vi "34970A Trigger+Read SW Scan v7.vi"(0 "VISA session":refnum<visa-resource-name>, 11 "error in":errorcluster, 12 "# Chan/Scan":i32, 13 "Error Query?":bool, 14 "Read delay mS":u32=1000) -> (4 "VISA out":refnum<visa-resource-name>, 6 "Strings":string[](array[string]), 8 "Pressures":T1, 10 "DBL":dbl[](array[numeric]) format="%.2f", 15 "error":errorcluster)   [LabVIEW 2020]
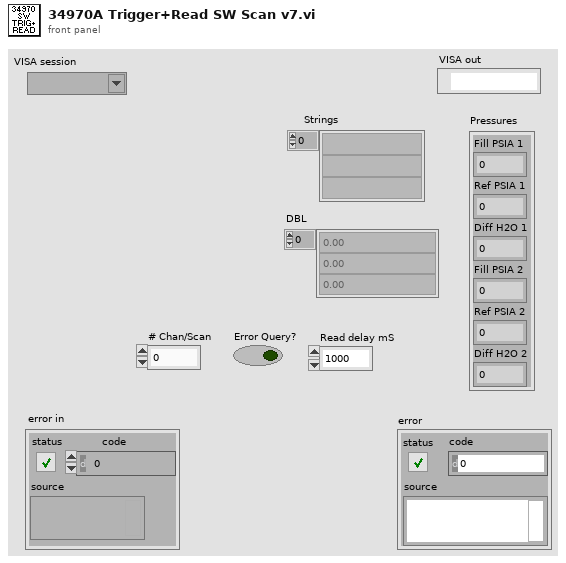
[diagram p1: front panel]
types:
  T1 = cluster{"Fill PSIA 1":dbl, "Ref PSIA 1":dbl, "Diff H2O 1":dbl, "Fill PSIA 2":dbl, "Ref PSIA 2":dbl, "Diff H2O 2":dbl}
  T2 = enum16{"Remote Trigger", "Immediate Trigger", "Wait for Trigger", "Abort Scan"}
  T3 = cluster{"Output Number Array[0]":dbl, "Output Number Array[1]":dbl, "Output Number Array[2]":dbl, "Output Number Array[3]":dbl, "Output Number Array[4]":dbl, "Output Number Array[5]":dbl}
  T4 = cluster{"Output Number Array[0]":dbl, "Output Number Array[1]":dbl, dbl, "Output Number Array[3]":dbl, "Output Number Array[4]":dbl, dbl}
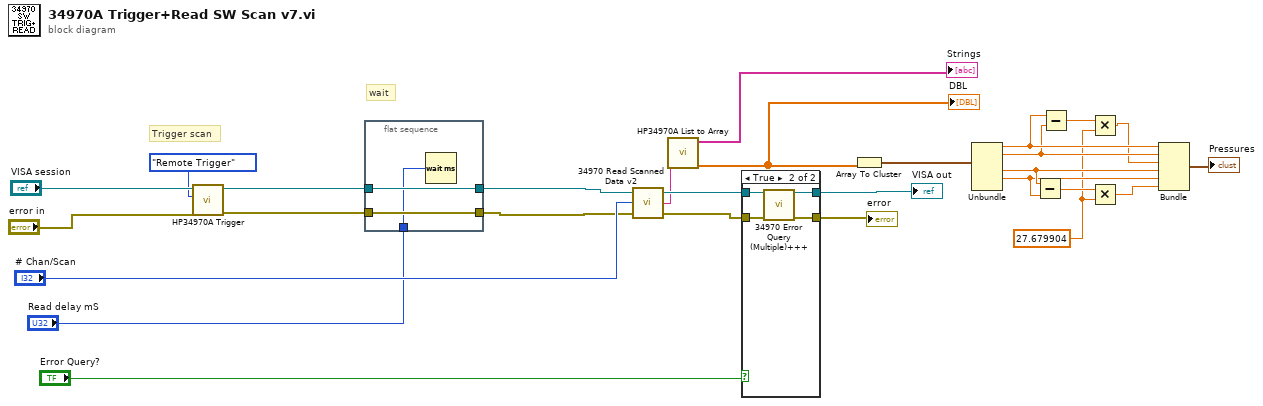
[diagram p0: block diagram]
diagram:
  w7 = 27.679904
  # "wait"
  # "Trigger scan"
  n1 = call "HP34970A Trigger.vi"("error in (no error)"="error in", "Command (0:Rem Trig)"=T2."Remote Trigger", "VISA session"="VISA session") -> ("error out"=w3:errorcluster, "dup VISA session"=w24:refnum<visa-resource-name>)  [unwired: 6 in]
  n2 = flat-sequence {
    tunnel: w24 -> [w31]
    tunnel: [w31] -> w19
    tunnel: [w30] -> w2
    tunnel: w3 -> [w30]
    tunnel: "Read delay mS" -> [w29]
    frame #0 {
      n3 = Wait (ms)(milliseconds to wait=w29) -> ()  [unwired: 1 out]
    }
  }
  n4 = call "34970 Read Scanned Data v2.vi"("error out"=w2, "# Channels"="# Chan/Scan", "VISA session 2"=w19) -> ("error"=w23:errorcluster, "Data String"=w18:string, "VISA Resource Name"=w22:refnum<visa-resource-name>)
  n5 = call "HP34970A List to Array.vi"("List (empty)"=w18) -> ("Output Number Array"=w5:dbl[], "Output String Array"=→"Strings":string[])  [unwired: 5 in]
  "DBL" <- w5
  n6 = case shown="True" "Error Query?" {
    tunnel: [w33 w37] -> w25
    tunnel: [w32 w36] -> w1
    tunnel: w23 -> [w32 w35]
    tunnel: w22 -> [w33 w34]
    frame False {
    }
    frame True {
      n7 = call "34970 Error Query (Multiple)+++.vi"("VISA resource name"=w34, "error in (no error)"=w35) -> ("VISA resource name out"=w37:refnum<visa-resource-name>, "error out"=w36:errorcluster)  [unwired: 10 in, 2 out]
    }
  }
  "error" <- w1
  "VISA out" <- w25
  n8 = Array To Cluster(array=w5) -> (cluster=w6:T3)
  n9 = Unbundle(w6) -> ("Output Number Array[0]"=w13:dbl, "Output Number Array[1]"=w12:dbl, "Output Number Array[3]"=w16:dbl, "Output Number Array[4]"=w15:dbl)  [unwired: 2 out]
  n10 = Subtract(x=w16, y=w15) -> (x-y=w10:dbl)
  n11 = Subtract(x=w13, y=w12) -> (x-y=w11:dbl)
  n12 = Multiply(x=w11, y=w7) -> (x*y=w8:dbl)
  n13 = Multiply(x=w10, y=w7) -> (x*y=w9:dbl)
  n14 = Bundle("Output Number Array[0]"=w13, "Output Number Array[1]"=w12, w8, "Output Number Array[3]"=w16, "Output Number Array[4]"=w15, w9) -> (→"Pressures":T4)  [unwired: 1 in]
